vi "notifyObservers.vi"(8 "error in (no error)":errorcluster, 11 "Observable in":refnum<class "Observable.lvclass">) -> (0 "error out":errorcluster, 3 "Observable out":refnum<class "Observable.lvclass">)   [LabVIEW 2018, in "Observable.lvclass"]
uses:
  Observable.lvclass
  Observer/Observer.lvclass
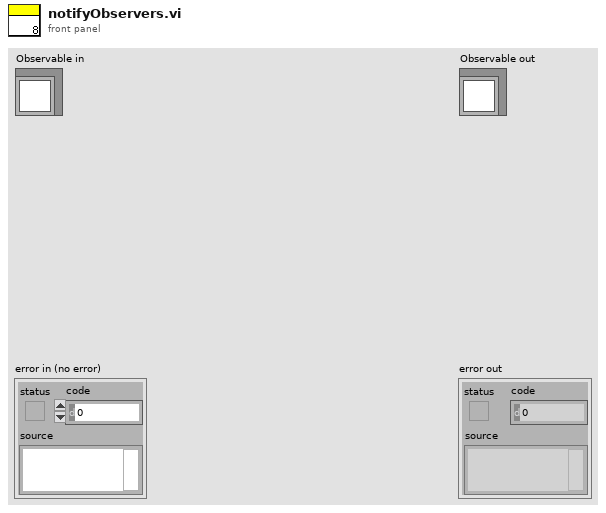
[diagram p1: front panel]
types:
  T1 = cluster{"Temperature":dbl, "Humidity":dbl, "Pressure":dbl, "Stop?":bool}
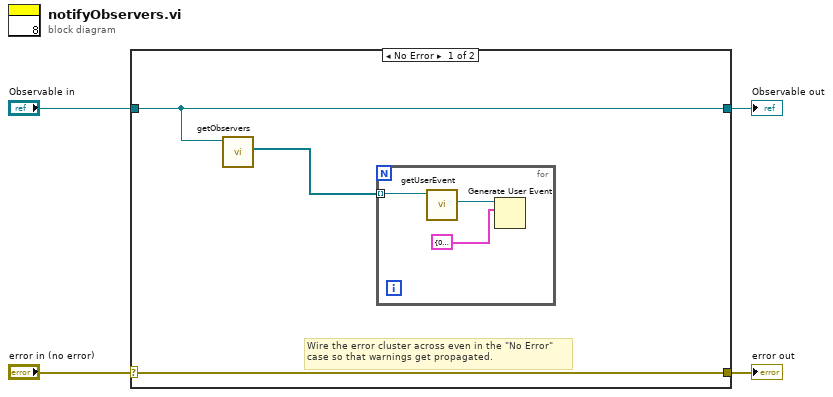
[diagram p0: block diagram]
diagram:
  n1 = case shown="No Error" "error in (no error)" {
    selector: "error in (no error)" -> [w7 w12]
    tunnel: [w7 w12] -> w3
    tunnel: [w5 w11] -> w1
    tunnel: "Observable in" -> [w5 w11]
    frame No Error {
      # "Wire the error cluster across even in the \"No Error\"\ncase so that warnings get propagated."
      n2 = call-dynamic "getObservers.vi"("Observable in"=w5) -> ("Observers"=w6:refnum<class "Observer.lvclass">[])  [unwired: 8 in, 2 out]
      n3 = for {
        tunnel: w6 -> [w10] mode=indexing
        n4 = call-dynamic "getUserEvent.vi"("Observer in"=w10) -> ("UserEvent"=w9:refnum<user-event>)  [unwired: 8 in, 2 out]
        n5 = Generate User Event(user event=w9, event data cluster=T1 {"Temperature"=0.0, "Humidity"=0.0, "Pressure"=0.0, "Stop?"=FALSE} ("event data")) -> ()  [unwired: 2 in, 2 out]
      }
    }
    frame Error {
    }
  }
  "error out" <- w3
  "Observable out" <- w1
